vi "CODMn微站质控流程 (子VI).vi"(10 "CODMn量程切换":enum32{"H", "L", "AUTO"}(ring)=enum."AUTO", 11 "COD":bool) -> (2 "CODMn中断报警":bool, 3 "布尔":bool)   [LabVIEW 2016, in "质控单元.lvlib"]
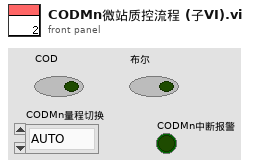
[diagram p1: front panel]
types:
  T1 = enum16{"待机", "启动水样测量", "水样测量中", "启动加标", "启动加标回收", "加标回收测量中", "结束"}
  T2 = cluster{"测量模式":enum16{"水样测量", "标样核查", "零点核查", "跨度核查", "空白测试", "加标回收", "平行样", "校零", "校标"}}
  T3 = enum16{"空闲", "水样测试", "标样核查", "零点核查", "跨度核查", "空白测试", "平行样测试", "质控样", "空白校准", "标样校准", "加标回收"}
  T4 = enum16{"空闲", "水样测试", "标样核查", "零点核查", "跨度核查", "空白测试", "平行样测试", "加标回收", "空白校准", "标样校准", "初始化（清洗）"}
  T5 = cluster{"量程":dbl, "检出限":dbl, "加标前水样浓度":dbl, "加标后水样浓度":dbl, "加标水杯定容体积":dbl, "加标母液浓度":dbl, "加标体积":dbl, "加标回收率":dbl}
  T6 = cluster{"氨氮":u8, "总磷":u8, "总氮":u8, "CODMn":u8, "CODCr":u8}
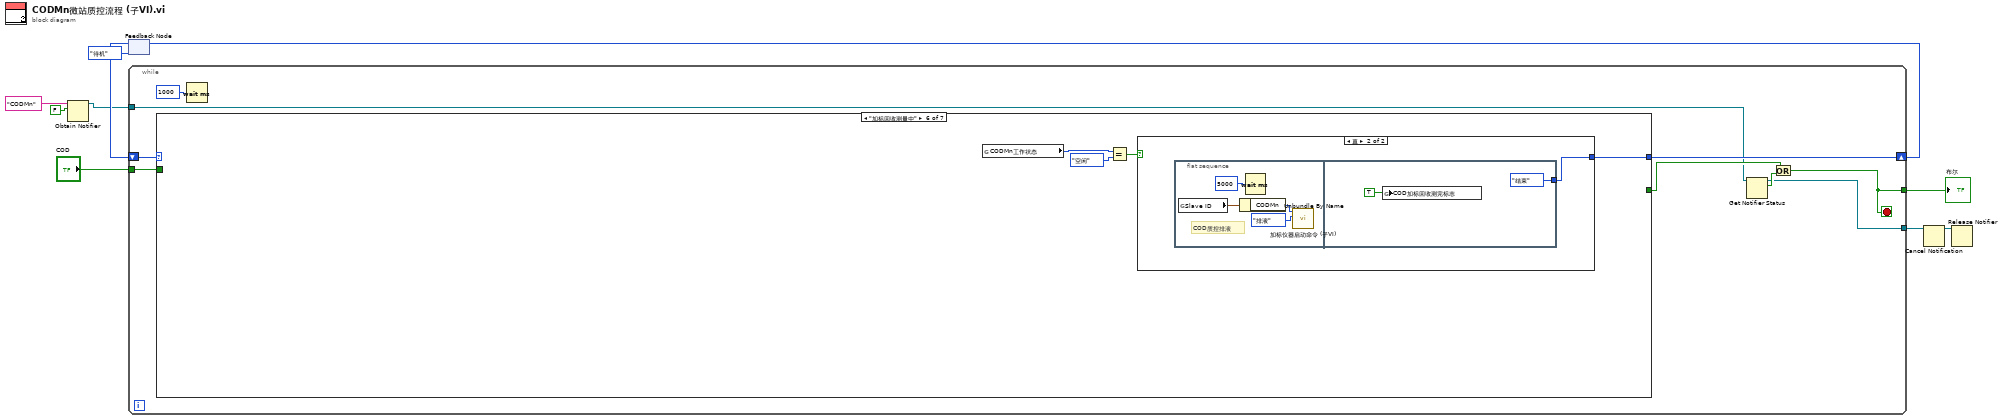
[diagram p0: block diagram]
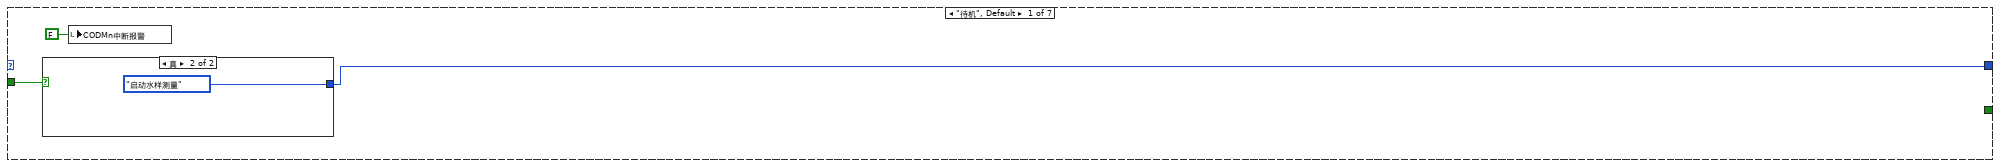
[diagram p2: hidden frame]
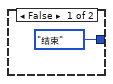
[diagram p3: hidden frame]
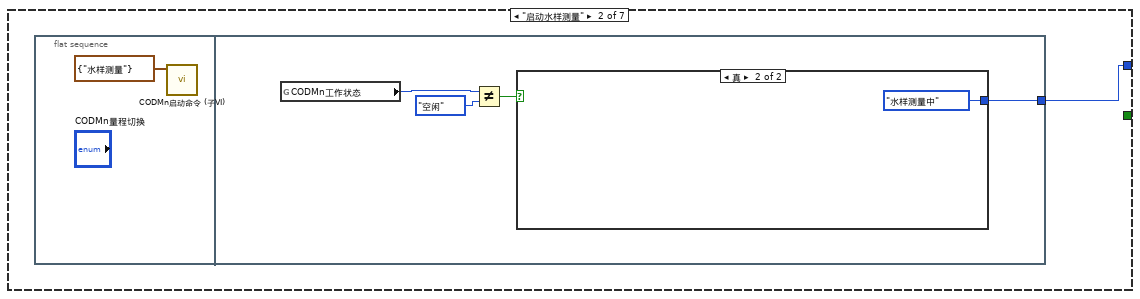
[diagram p4: hidden frame]
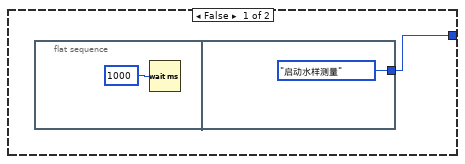
[diagram p5: hidden frame]
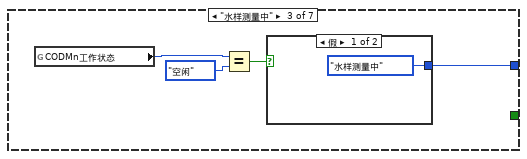
[diagram p6: hidden frame]
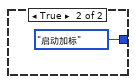
[diagram p7: hidden frame]
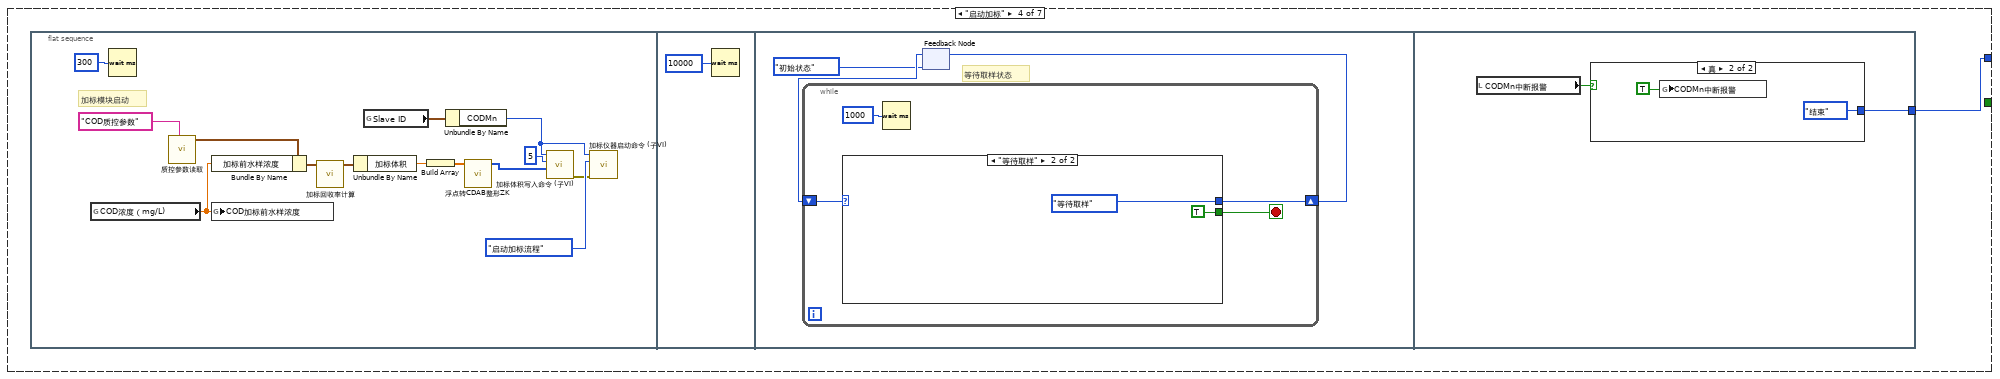
[diagram p8: hidden frame]
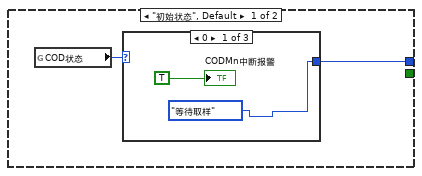
[diagram p9: hidden frame]
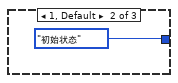
[diagram p10: hidden frame]
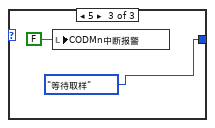
[diagram p11: hidden frame]
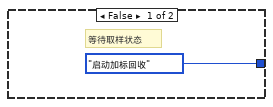
[diagram p12: hidden frame]
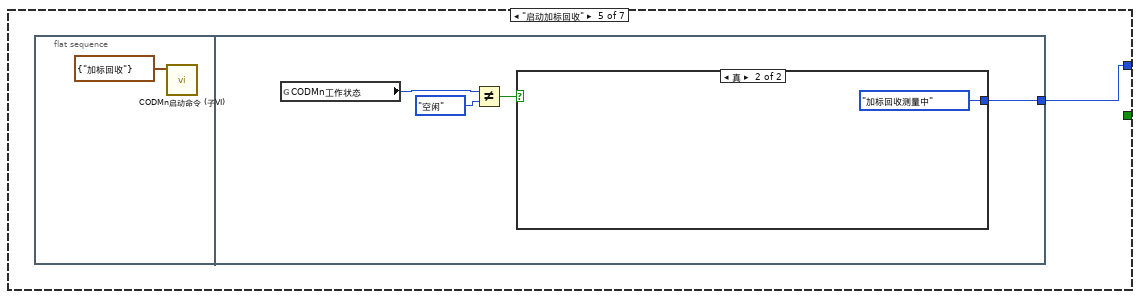
[diagram p13: hidden frame]
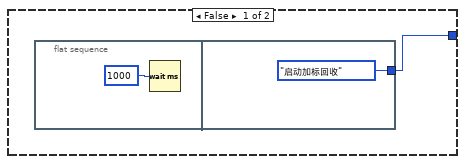
[diagram p14: hidden frame]
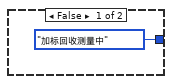
[diagram p15: hidden frame]
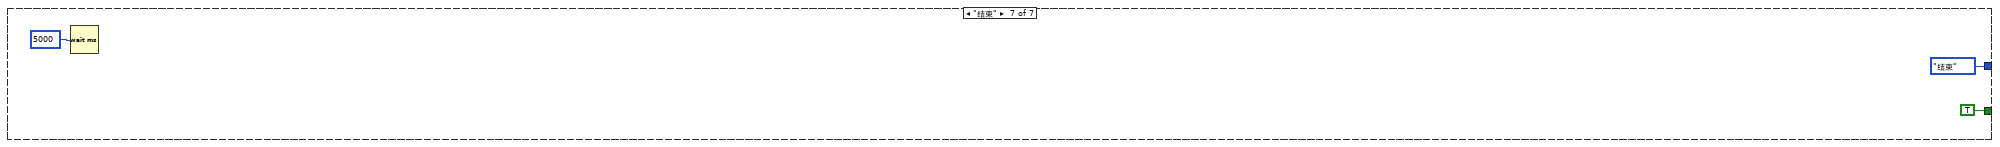
[diagram p16: hidden frame]
diagram:
  n1 = Obtain Notifier(name (unnamed)="CODMn" ("名称（未命名）"), notification data type=FALSE) -> (notifier out=w1:refnum<notifier>)  [unwired: 2 in, 2 out]
  n2 = feedback #1(T1."待机") -> (w6:T1)
  n3 = while {
    tunnel: "COD" -> [w19]
    tunnel: [w14] -> w8
    shift-right: [w18] -> w9
    shift-left: w6 -> [w16]
    tunnel: [w12] -> w2
    tunnel: w1 -> [w11]
    stop <- w14 stop-if-true
    n4 = case shown="\"加标回收测量中\"" w16 {
      tunnel: [w22 w25 w38 w41 w78 w91 T1."结束"] -> w18
      tunnel: [_ _ _ _ _ _ TRUE] -> w13
      tunnel: w19 -> [w21 _ _ _ _ _ _]
      frame "待机", Default {
        n5 = case shown="真" w21 {
          tunnel: [T1."结束" T1."启动水样测量"] -> w22
          frame False {
          }
          frame True {
          }
        }
        n6 = local write "CODMn中断报警"(FALSE ("CODMn中断报警")) -> ()
      }
      frame "启动水样测量" {
        n7 = flat-sequence {
          tunnel: [w30] -> w25
          frame #0 {
            n8 = call "CODMn启动命令 (子VI).vi"("启动测量模式"=T2 {"测量模式"=enum."水样测量"}) -> ()  [unwired: 10 in, 1 out]
          }
          frame #1 {
            n9 = global read "与CODMn交互全局.vi" "CODMn工作状态"() -> (w29:T4)
            n10 = Not Equal?(x=w29, y=T3."空闲") -> (x != y?=w27:bool)
            n11 = case shown="真" w27 {
              tunnel: [w31 T1."水样测量中"] -> w30
              frame False {
                n12 = flat-sequence {
                  tunnel: [T1."启动水样测量"] -> w31
                  frame #0 {
                    n13 = Wait (ms)(milliseconds to wait=u32 1000 ("等待时间（毫秒）")) -> ()  [unwired: 1 out]
                  }
                  frame #1 {
                  }
                }
              }
              frame True {
              }
            }
          }
        }
      }
      frame "水样测量中" {
        n14 = global read "与CODMn交互全局.vi" "CODMn工作状态"() -> (w37:T4)
        n15 = Equal?(x=w37, y=T3."空闲") -> (x = y?=w35:bool)
        n16 = case shown="假" w35 {
          tunnel: [T1."水样测量中" T1."启动加标"] -> w38
          frame False {
          }
          frame True {
          }
        }
      }
      frame "启动加标" {
        n17 = flat-sequence {
          tunnel: [w74] -> w41
          frame #0 {
            # "加标模块启动"
            n18 = global read "与CODMn交互全局.vi" "COD浓度（mg/L)"() -> (w49:dbl)
            n19 = Wait (ms)(milliseconds to wait=u32 300 ("等待时间（毫秒）")) -> ()  [unwired: 1 out]
            n20 = call "质控参数读取.vi"("section"="COD质控参数") -> ("参数"=w53:T5)  [unwired: 9 in, 1 out]
            n21 = Bundle By Name(cluster=w53, "加标前水样浓度"=w49) -> (w54:T5)
            n22 = global write "水样浓度全局.vi" "COD加标前水样浓度"(w49) -> ()
            n23 = call "加标回收率计算.vi"("参数"=w54) -> ("参数 out"=w52:T5)  [unwired: 9 in, 1 out]
            n24 = Unbundle By Name(w52) -> ("加标体积"=w50:dbl)
            n25 = global read "断电保存全局.vi" "Slave ID"() -> (w43:T6)
            n26 = Build Array(w50) -> (w51:dbl[])
            n27 = Unbundle By Name(w43) -> ("CODMn"=w42:u8)
            n28 = call "浮点转CDAB整形ZK.vi"("浮点数"=w51) -> ("CDAB整形输出"=w44:u16[])  [unwired: 10 in]
            n29 = call "加标体积写入命令 (子VI).vi"("values"=w44, "starting address"=u16 5, "Slave ID"=w42) -> ("错误输出"=w45:errorcluster)  [unwired: 8 in]
            n30 = call "加标仪器启动命令 (子VI).vi"("错误输入（无错误）"=w45, "启动命令"=enum16{"启动水样流程", "启动加标流程", "排液", "停止"}."启动加标流程", "仪器"=w42) -> ()  [unwired: 8 in, 1 out]
          }
          frame #1 {
            n31 = Wait (ms)(milliseconds to wait=u32 10000 ("等待时间（毫秒）")) -> ()  [unwired: 1 out]
          }
          frame #2 {
            # "等待取样状态"
            n32 = feedback #2(enum16{"初始状态", "等待取样"}."初始状态") -> (w59:enum16{"初始状态", "等待取样"})
            n33 = while {
              shift-right: [w62] -> w58
              shift-left: w59 -> [w63]
              stop <- w61 stop-if-true
              n34 = case shown="\"等待取样\"" w63 {
                tunnel: [w65 enum16{"初始状态", "等待取样"}."等待取样"] -> w62
                tunnel: [_ TRUE] -> w61
                frame "初始状态", Default {
                  n35 = global read "加标回收状态全局变量.vi" "COD状态"() -> (w64:u16)
                  n36 = case shown="0" w64 {
                    tunnel: [enum16{"初始状态", "等待取样"}."等待取样" enum16{"初始状态", "等待取样"}."初始状态" enum16{"初始状态", "等待取样"}."等待取样"] -> w65
                    frame 0 {
                      "CODMn中断报警" <- TRUE ("CODMn中断报警")
                    }
                    frame 1, Default {
                    }
                    frame 5 {
                      n37 = local write "CODMn中断报警"(FALSE ("CODMn中断报警")) -> ()
                    }
                  }
                }
                frame "等待取样" {
                }
              }
              n38 = Wait (ms)(milliseconds to wait=u32 1000 ("等待时间（毫秒）")) -> ()  [unwired: 1 out]
            }
            n39 = feedback-in #2(w58) -> ()
          }
          frame #3 {
            n40 = local read "CODMn中断报警"() -> (w73:bool)
            n41 = case shown="真" w73 {
              tunnel: [T1."启动加标回收" T1."结束"] -> w74
              frame False {
                # "等待取样状态"
              }
              frame True {
                n42 = global write "质控中断报警全局.vi" "CODMn中断报警"(TRUE ("CODMn中断报警")) -> ()
              }
            }
          }
        }
      }
      frame "启动加标回收" {
        n43 = flat-sequence {
          tunnel: [w83] -> w78
          frame #0 {
            n44 = call "CODMn启动命令 (子VI).vi"("启动测量模式"=T2 {"测量模式"=enum."加标回收"}) -> ()  [unwired: 10 in, 1 out]
          }
          frame #1 {
            n45 = global read "与CODMn交互全局.vi" "CODMn工作状态"() -> (w82:T4)
            n46 = Not Equal?(x=w82, y=T3."空闲") -> (x != y?=w80:bool)
            n47 = case shown="真" w80 {
              tunnel: [w84 T1."加标回收测量中"] -> w83
              frame False {
                n48 = flat-sequence {
                  tunnel: [T1."启动加标回收"] -> w84
                  frame #0 {
                    n49 = Wait (ms)(milliseconds to wait=u32 1000 ("等待时间（毫秒）")) -> ()  [unwired: 1 out]
                  }
                  frame #1 {
                  }
                }
              }
              frame True {
              }
            }
          }
        }
      }
      frame "加标回收测量中" {
        n50 = global read "与CODMn交互全局.vi" "CODMn工作状态"() -> (w90:T4)
        n51 = Equal?(x=w90, y=T3."空闲") -> (x = y?=w88:bool)
        n52 = case shown="真" w88 {
          tunnel: [T1."加标回收测量中" w93] -> w91
          frame False {
          }
          frame True {
            n53 = flat-sequence {
              tunnel: [T1."结束"] -> w93
              frame #0 {
                # "COD质控排液"
                n54 = global read "断电保存全局.vi" "Slave ID"() -> (w95:T6)
                n55 = Unbundle By Name(w95) -> ("CODMn"=w94:u8)
                n56 = Wait (ms)(milliseconds to wait=u32 5000 ("等待时间（毫秒）")) -> ()  [unwired: 1 out]
                n57 = call "加标仪器启动命令 (子VI).vi"("启动命令"=enum16{"启动水样流程", "启动加标流程", "排液", "停止"}."排液", "仪器"=w94) -> ()  [unwired: 9 in, 1 out]
              }
              frame #1 {
                n58 = global write "质控测完标志全局 1.vi" "COD加标回收测完标志"(TRUE ("COD加标回收测完标志")) -> ()
              }
            }
          }
        }
      }
      frame "结束" {
        n59 = Wait (ms)(milliseconds to wait=u32 5000 ("等待时间（毫秒）")) -> ()  [unwired: 1 out]
      }
    }
    n60 = Wait (ms)(milliseconds to wait=u32 1000 ("等待时间（毫秒）")) -> ()  [unwired: 1 out]
    n61 = Get Notifier Status(notifier=w11) -> (notifier out=w12:refnum<notifier>, current notification=w15:bool)  [unwired: 1 in, 3 out]
    n62 = Or(x=w13, y=w15) -> (x .or. y?=w14:bool)
  }
  "布尔" <- w8
  n63 = feedback-in #1(w9) -> ()
  n64 = Cancel Notification(0:w2) -> (8:w3:refnum<notifier>)  [unwired: 1 in, 2 out]
  n65 = Release Notifier(notifier=w3) -> ()  [unwired: 2 in, 3 out]
